vi "Respond with Devices for Measurement.vi"(6 "Measurement Name":string, 8 "error in (no error)":errorcluster, 9 "Hardware Type":string, 10 "Matching Devices":string[](array[string]), 11 "Controller in":refnum<class "Controller.lvclass">) -> (0 "error out":errorcluster, 3 "Controller out":refnum<class "Controller.lvclass">)   [LabVIEW 2017, in "Controller Actor.lvlib" / "Controller.lvclass"]
uses:
  Controller.lvclass
  Msmt UI/Messages/Display Hardware Devices Msg/Display Hardware Devices Msg.lvclass/Display Hardware Devices Msg.ctl
  <vilib>/ActorFramework/Message Enqueuer/Message Enqueuer.lvclass/Message Enqueuer.ctl
  <vilib>/ActorFramework/Message Enqueuer/Enqueue.vi
  Msmt UI/Messages/Display Hardware Devices Msg/Display Hardware Devices Msg.lvclass
  C:/Program Files (x86)/National Instruments/LabVIEW 2017/vi.lib/ActorFramework/Message/Message.lvclass
  <vilib>/ActorFramework/Message Priority Queue/Priority Enqueue.vi
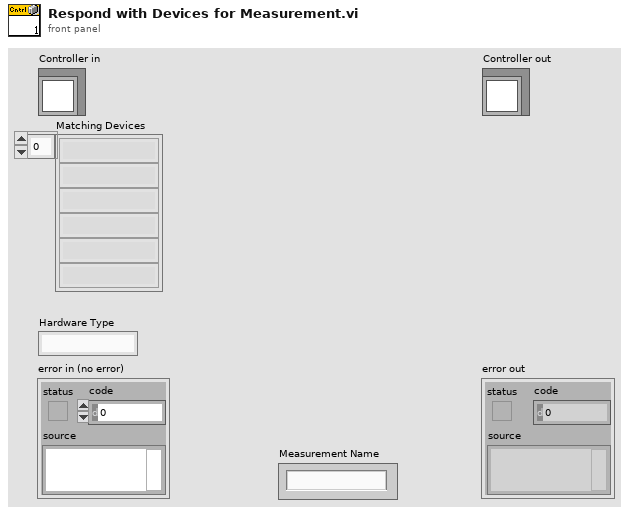
[diagram p1: front panel]
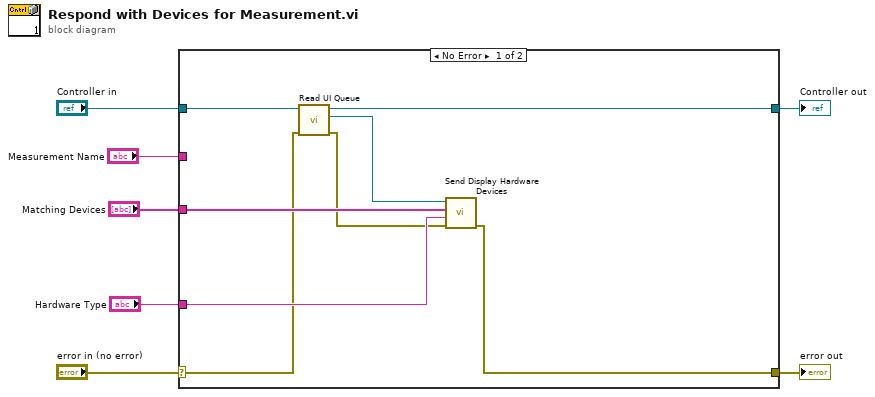
[diagram p0: block diagram]
diagram:
  n1 = case shown="No Error" "error in (no error)" {
    selector: "error in (no error)" -> [w9 w17]
    tunnel: [w8 w17] -> w6
    tunnel: [w11 w16] -> w4
    tunnel: "Controller in" -> [w12 w16]
    tunnel: "Matching Devices" -> [w14 _]
    tunnel: "Hardware Type" -> [w15 _]
    tunnel: "Measurement Name" -> [_ _]
    frame No Error {
      n2 = call "Read UI Queue.vi"("error in (no error)"=w9, "UI Controller in"=w12) -> ("error out"=w10:errorcluster, "UI Queue"=w13:refnum<class "Message Enqueuer.lvclass">, "UI Controller out"=w11:refnum<class "Controller.lvclass">)  [unwired: 7 in]
      n3 = call "Send Display Hardware Devices.vi"("error in (no error)"=w10, "Hardware Type"=w15, "Array of Hardware Device Names"=w14, "Message Enqueuer"=w13) -> ("error out"=w8:errorcluster)  [unwired: 6 in, 1 out]
    }
    frame Error {
    }
  }
  "error out" <- w6
  "Controller out" <- w4
